vi "Find All 429 Channels on Card.vi"(0 "Card Number":i32, 11 "error in (no error)":errorcluster) -> (3 "Core Numbers":i32[](array[numeric]), 4 "Number of RX Channels":i32[](array[numeric]), 6 "Rx Channels":i32[][](array[numeric]), 8 "Number of TX Channels":i32[](array[numeric]), 10 "Tx Channels":i32[][](array[numeric]), 15 "error out":errorcluster)   [LabVIEW 2019]
doc: "This program opens the specified card, then searches through 4 possible cores for valid 429 Receive and Transmit Channels. The list of valid Core Numbers is returned in an array. The list of valid Channel numbers are returned in 2 two-dimensional arrays."
uses:
  <instrlib>/BTICardLib/Private/Initialize By Card Number and Core Number.vi
  <instrlib>/BTICardLib/BTICardLV.lvlib
  <instrlib>/BTI429Lib/BTI429LV.lvlib
panel:
  # "ARINC 429: Find All 429 Channels on Card"
  # "©2016 Astronics Ballard Technology"
  # "This program opens the specified card, then searches through 4 possible cores for valid 429 Receive and Transmit Channels. The list of valid Core Numbers is returned in an array. The list of valid Channel numbers are returned in 2 two-dimensional arrays."
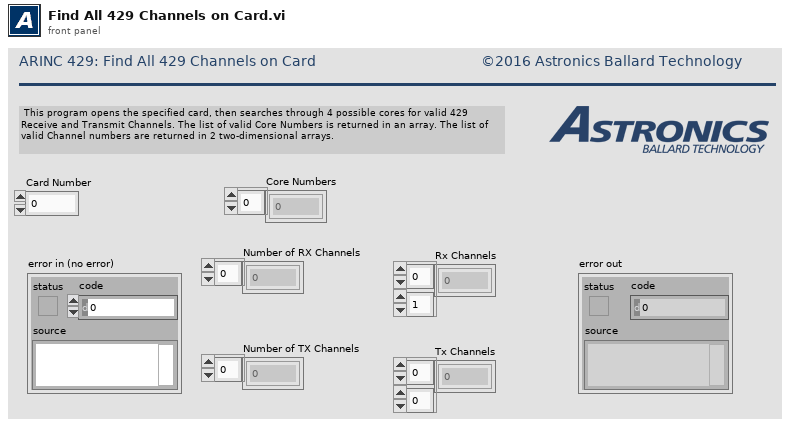
[diagram p1: front panel]
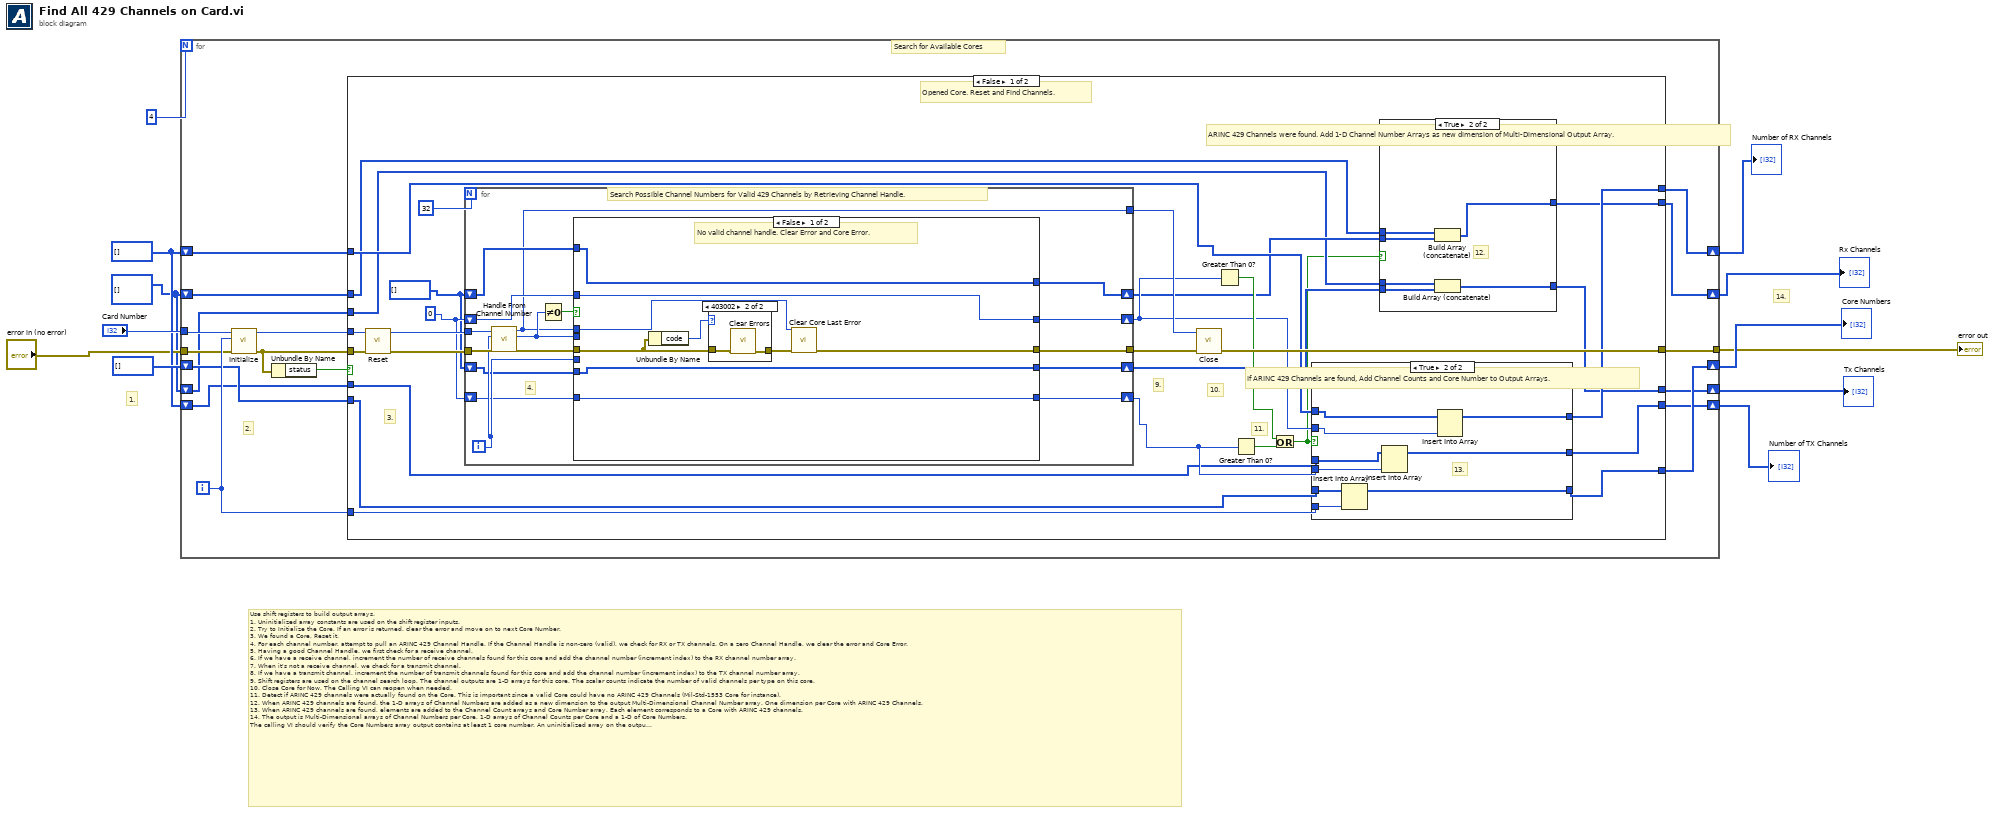
[diagram p0: block diagram]
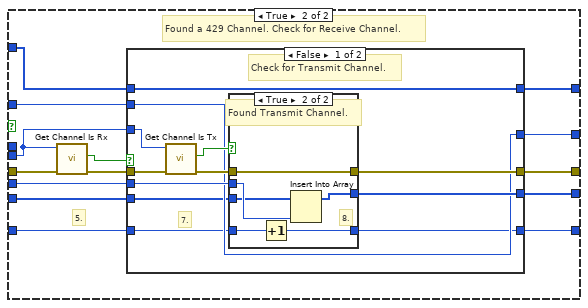
[diagram p5: hidden frame]
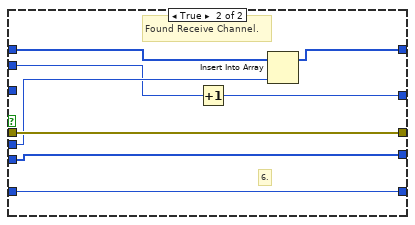
[diagram p7: hidden frame]
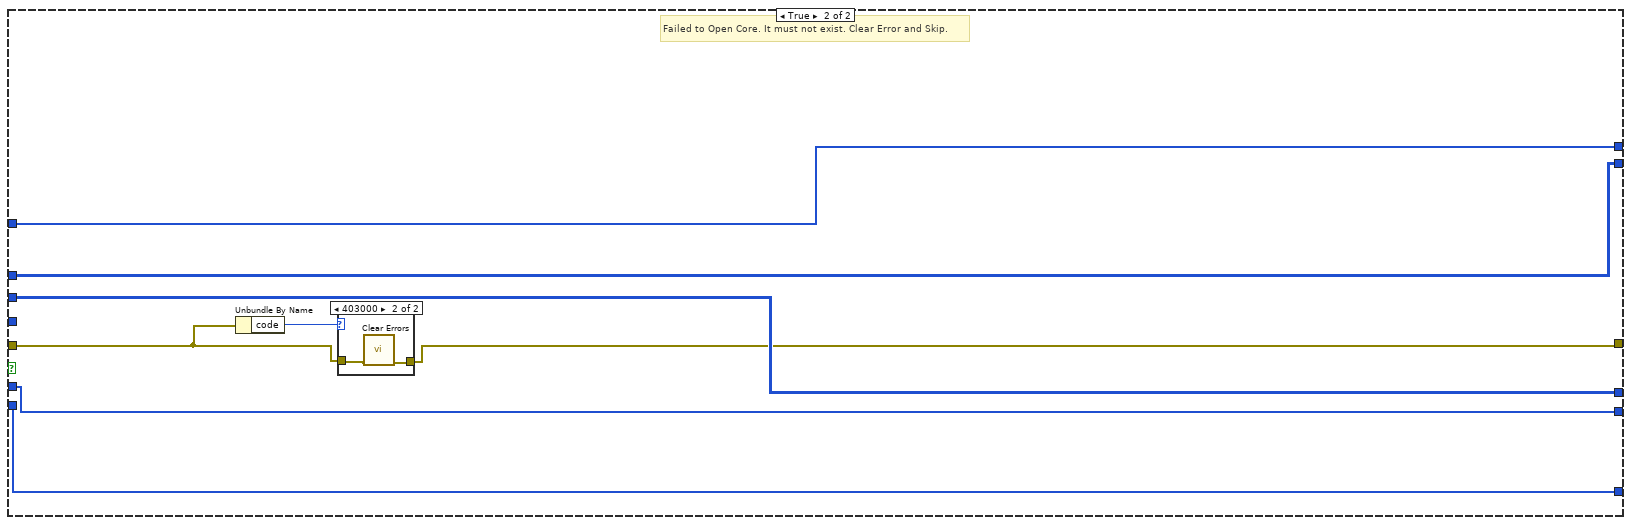
[diagram p8: hidden frame]
diagram:
  w3 = i32[][] [] ("channel handle out")
  w5 = i32[] []
  # "14."
  # "1."
  # "Use shift registers to build output arrays.\n1. Uninitialized array constants are used on the shift register inputs.\n2. Try to Initialize the Core. If an error is returned, clear the error and move on to next Core Number.\n3. We found a Core, Reset it.\n4. For each channel number, attempt to pull an ARINC 429 Channel Handle. If the Channel Handle is non-zero (valid), we check for RX or TX channels. On a zero Channel Handle, we clear the error and Core Error.\n5. Having a good Channel Handle, we first check for a receive channel.\n6. If we have a receive channel, increment the number of receive channels found for this core and add the channel number (increment index) to the RX channel number array.\n7. When it's not a receive channel, we check for a transmit channel.\n8. If we have a transmit channel, increment the number of transmit channels found for this core and add the channel number (increment index) to the TX channel number array.\n9. Shift registers are used on the channel search loop. The channel outputs are 1-D arrays for this core. The scalar counts indicate the number of valid channels per type on this core.\n10. Close Core for Now. The Calling VI can reopen when needed. \n11. Detect if ARINC 429 channels were actually found on the Core. This is important since a valid Core could have no ARINC 429 Channels (Mil-Std-1553 Core for instance).\n12. When ARINC 429 channels are found, the 1-D arrays of Channel Numbers are added as a new dimension to the output Multi-Dimensional Channel Number array. One dimension per Core with ARINC 429 Channels.\n13. When ARINC 429 channels are found, elements are added to the Channel Count arrays and Core Number array. Each element corresponds to a Core with ARINC 429 channels.\n14. The output is Multi-Dimensional arrays of Channel Numbers per Core, 1-D arrays of Channel Counts per Core and a 1-D of Core Numbers.\nThe calling VI should verify the Core Numbers array output contains at least 1 core number. An uninitialized array on the output means no ARINC 429 cores/channels were found on the specified device."
  n1 = for {
    N: 4 -> [_]
    tunnel: "Card Number" -> [w29]
    tunnel: [w25] -> w9
    shift-right: [w20] -> w10
    shift-left: i32[] [] -> [w23]
    shift-right: [w22] -> w7
    shift-left: w5 -> [w21]
    shift-right: [w19] -> w6
    shift-left: w5 -> [w18]
    tunnel: "error in (no error)" -> [w17]
    shift-right: [w13] -> w1
    shift-left: w3 -> [w14]
    shift-right: [w15] -> w2
    shift-left: w3 -> [w16]
    i -> [w24]
    # "2."
    # "Search for Available Cores"
    n2 = call-poly <instrlib>:"Initialize.vi"("error in (no error)"=w17, "core number"=w24, "card number"=w29) -> ("error out"=w26:errorcluster, "core handle out"=w27:u64)  [unwired: 7 in]
    n3 = Unbundle By Name(w26) -> ("status"=w28:bool)
    n4 = case shown="False" w28 {
      tunnel: w27 -> [w57 _]
      tunnel: w26 -> [w56 w150]
      tunnel: [w36 w153] -> w15
      tunnel: [w51 w149] -> w25
      tunnel: w24 -> [w49 _]
      tunnel: w23 -> [w48 w156]
      tunnel: [w38 w155] -> w22
      tunnel: w21 -> [w39 w155]
      tunnel: [w47 w156] -> w20
      tunnel: [w41 w154] -> w19
      tunnel: w18 -> [w42 w154]
      tunnel: w16 -> [w34 w153]
      tunnel: w14 -> [w31 w152]
      tunnel: [w32 w152] -> w13
      frame False {
        w35 = i32[] [] ("channel handle out")
        w46 = 0
        # "11."
        # "10."
        # "9."
        # "3."
        # "Opened Core. Reset and Find Channels."
        n5 = call <instrlib>:"Reset.vi"("error in (no error)"=w56, "core handle in"=w57) -> ("error out"=w54:errorcluster, "core handle out"=w53:u64)  [unwired: 8 in]
        n6 = for {
          N: 32 -> [_]
          tunnel: w54 -> [w93]
          tunnel: w53 -> [w92]
          tunnel: [w89] -> w52
          tunnel: [w78] -> w50
          shift-right: [w90] -> w37
          shift-left: w35 -> [w84]
          shift-right: [w83] -> w40
          shift-left: w46 -> [w82]
          shift-right: [w91] -> w33
          shift-left: w35 -> [w81]
          shift-right: [w80] -> w43
          shift-left: w46 -> [w79]
          i -> [w85]
          # "4."
          # "Search Possible Channel Numbers for Valid 429 Channels by Retrieving Channel Handle."
          n7 = call <instrlib>:"Handle From Channel Number.vi"("error in (no error)"=w93, "channel number"=w85, "core handle in"=w92) -> ("error out"=w88:errorcluster, "channel handle out"=w86:u64, "core handle out"=w78:u64)  [unwired: 6 in]
          n8 = Not Equal To 0?(x=w86) -> (x != 0?=w87:bool)
          n9 = case shown="False" w87 {
            tunnel: w86 -> [_ w117]
            tunnel: [w100 w116] -> w91
            tunnel: [w102 w115] -> w90
            tunnel: [w97 w114] -> w89
            tunnel: w88 -> [w95 w113]
            tunnel: w85 -> [_ w112]
            tunnel: w84 -> [w102 w111]
            tunnel: w82 -> [w101 w110]
            tunnel: [w101 w109] -> w83
            tunnel: w81 -> [w100 w108]
            tunnel: [w99 w107] -> w80
            tunnel: w79 -> [w99 w106]
            tunnel: w78 -> [w98 _]
            frame False {
              # "No valid channel handle. Clear Error and Core Error."
              n10 = Unbundle By Name(w95) -> ("code"=w94:i32)
              n11 = case shown="403002" w94 {
                tunnel: [w103 w105] -> w96
                tunnel: w95 -> [w103 w104]
                frame Default {
                }
                frame 403002 {
                  n12 = call <vilib>:"Clear Errors.vi"("error in (no error)"=w104) -> ("error out"=w105:errorcluster)  [unwired: 5 in, 1 out]
                }
              }
              n13 = call <instrlib>:"Clear Core Last Error.vi"("error in (no error)"=w96, "handle in"=w98) -> ("error out"=w97:errorcluster)  [unwired: 8 in, 1 out]
            }
            frame True {
              # "5."
              # "Found a 429 Channel. Check for Receive Channel."
              n14 = call <instrlib>:"Get Channel Is Rx.vi"("error in (no error)"=w113, "channel handle in"=w117) -> ("error out"=w118:errorcluster, "channel is receive?"=w119:bool)  [unwired: 7 in, 1 out]
              n15 = case shown="False" w119 {
                tunnel: w118 -> [w126 w148]
                tunnel: [w128 w148] -> w114
                tunnel: [w127 w142] -> w116
                tunnel: w117 -> [w131 _]
                tunnel: [w124 w147] -> w115
                tunnel: w112 -> [w125 w145]
                tunnel: w111 -> [w124 w146]
                tunnel: w110 -> [w123 w144]
                tunnel: [w123 w143] -> w109
                tunnel: w108 -> [w122 w142]
                tunnel: [w121 w141] -> w107
                tunnel: w106 -> [w120 w141]
                frame False {
                  # "7."
                  # "Check for Transmit Channel."
                  n16 = call <instrlib>:"Get Channel Is Tx.vi"("error in (no error)"=w126, "channel handle in"=w131) -> ("error out"=w129:errorcluster, "channel is transmit?"=w130:bool)  [unwired: 7 in, 1 out]
                  n17 = case shown="True" w130 {
                    tunnel: w129 -> [w134 w140]
                    tunnel: [w134 w140] -> w128
                    tunnel: [w133 w138] -> w127
                    tunnel: w125 -> [_ w139]
                    tunnel: w122 -> [w133 w137]
                    tunnel: [w132 w136] -> w121
                    tunnel: w120 -> [w132 w135]
                    frame False {
                      # "Not a Transmit Channel."
                    }
                    frame True {
                      # "8."
                      # "Found Transmit Channel."
                      n18 = Increment(x=w135) -> (x+1=w136:i32)
                      n19 = Insert Into Array(array=w137, new element=w139) -> (w138:i32[])  [unwired: 1 in]
                    }
                  }
                }
                frame True {
                  # "6."
                  # "Found Receive Channel."
                  n20 = Increment(x=w144) -> (x+1=w143:i32)
                  n21 = Insert Into Array(array=w146, new element=w145) -> (w147:i32[])  [unwired: 1 in]
                }
              }
            }
          }
        }
        n22 = call <instrlib>:"Close.vi"("error in (no error)"=w52, "core handle in"=w50) -> ("error out"=w51:errorcluster)  [unwired: 8 in, 1 out]
        n23 = Greater Than 0?(x=w40) -> (x > 0?=w44:bool)
        n24 = Greater Than 0?(x=w43) -> (x > 0?=w45:bool)
        n25 = Or(x=w44, y=w45) -> (x .or. y?=w30:bool)
        n26 = case shown="True" w30 {
          tunnel: w49 -> [_ w77]
          tunnel: w48 -> [w68 w76]
          tunnel: [w68 w75] -> w47
          tunnel: w43 -> [_ w74]
          tunnel: w42 -> [w67 w73]
          tunnel: [w67 w72] -> w41
          tunnel: w40 -> [_ w71]
          tunnel: w39 -> [w66 w70]
          tunnel: [w66 w69] -> w38
          frame False {
            # "No ARINC 429 Channels, so add nothing to output arrays for this core."
          }
          frame True {
            # "13."
            # "If ARINC 429 Channels are found, Add Channel Counts and Core Number to Output Arrays."
            n27 = Insert Into Array(array=w76, new element=w77) -> (w75:i32[])  [unwired: 1 in]
            n28 = Insert Into Array(array=w73, new element=w74) -> (w72:i32[])  [unwired: 1 in]
            n29 = Insert Into Array(array=w70, new element=w71) -> (w69:i32[])  [unwired: 1 in]
          }
        }
        n30 = case shown="True" w30 {
          tunnel: w37 -> [_ w65]
          tunnel: [w59 w64] -> w36
          tunnel: w34 -> [w59 w63]
          tunnel: w33 -> [_ w62]
          tunnel: [w58 w61] -> w32
          tunnel: w31 -> [w58 w60]
          frame False {
            # "No ARINC 429 Channels, so add nothing to output arrays for this core."
          }
          frame True {
            # "12."
            # "ARINC 429 Channels were found. Add 1-D Channel Number Arrays as new dimension of Multi-Dimensional Output Array."
            n31 = Build Array (concatenate)(w63, w65) -> (w64:i32[][])
            n32 = Build Array (concatenate)(w60, w62) -> (w61:i32[][])
          }
        }
      }
      frame True {
        # "Failed to Open Core. It must not exist. Clear Error and Skip."
        n33 = Unbundle By Name(w150) -> ("code"=w151:i32)
        n34 = case shown="403000" w151 {
          tunnel: [w157 w159] -> w149
          tunnel: w150 -> [w157 w158]
          frame Default {
          }
          frame 403000 {
            n35 = call <vilib>:"Clear Errors.vi"("error in (no error)"=w158) -> ("error out"=w159:errorcluster)  [unwired: 5 in, 1 out]
          }
        }
      }
    }
  }
  "Rx Channels" <- w2
  "Core Numbers" <- w10
  "Tx Channels" <- w1
  "error out" <- w9
  "Number of RX Channels" <- w7
  "Number of TX Channels" <- w6
